vi "CAN Read.vi"(8 "error in (no error)":errorcluster, 9 "TimestampBuffer":T1, 10 "MessageBuffer":T2, 11 "Channel":u16) -> (0 "error out":errorcluster, 1 "TimestampBuffer out":T1, 2 "MessageBuffer out":T2, 3 "function return":u32)   [LabVIEW 2021]
doc: "TPCANStatus __stdcall CAN_Read(\n TPCANHandle Channel, \n TPCANMsg* MessageBuffer, \n TPCANTimestamp* TimestampBuffer);"
uses:
  PCANBasic.dll
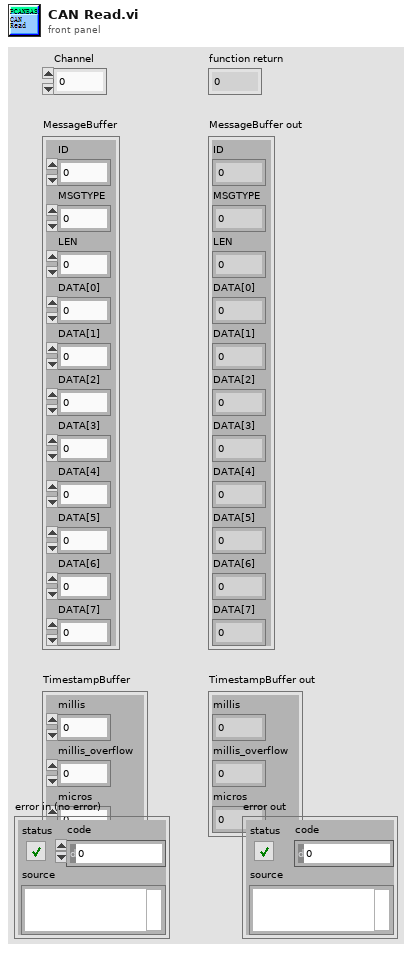
[diagram p1: front panel]
types:
  T1 = cluster{"millis":u32, "millis_overflow":u16, "micros":u16}
  T2 = cluster{"ID":u32, "MSGTYPE":u8, "LEN":u8, "DATA[0]":u8, "DATA[1]":u8, "DATA[2]":u8, "DATA[3]":u8, "DATA[4]":u8, "DATA[5]":u8, "DATA[6]":u8, "DATA[7]":u8}
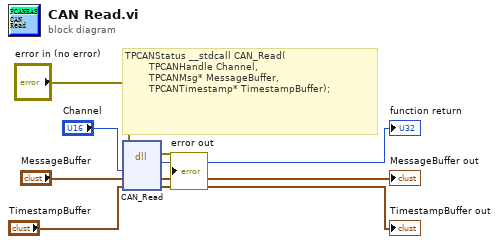
[diagram p0: block diagram]
diagram:
  # "TPCANStatus __stdcall CAN_Read(\n        TPCANHandle Channel, \n        TPCANMsg* MessageBuffer, \n        TPCANTimestamp* TimestampBuffer);"
  n1 = dll-call lib="PTH2_abs CUsersAdministrator.CH-202202160008Desktop传感器测试\tcan驱动PCANBasic.*" fn="CAN_Read"(error in="error in (no error)", "Channel"="Channel", "MessageBuffer"="MessageBuffer", "TimestampBuffer"="TimestampBuffer") -> (error out=→"error out":errorcluster, →"function return":u32, "MessageBuffer"=→"MessageBuffer out":T2, "TimestampBuffer"=→"TimestampBuffer out":T1)  [unwired: 3 in, 1 out]
